vi "Write Subordinate Object Queue.vi"(8 "error in (no error)":errorcluster, 9 "Name":string, 10 "Caller-To-Actor Enqueuer":refnum<class "Message Enqueuer.lvclass">, 11 "Measure Object in":refnum<class "Template Module.lvclass">) -> (0 "error out":errorcluster, 3 "Measure Object out":refnum<class "Template Module.lvclass">)   [LabVIEW 2018, in "Template Module.lvclass"]
uses:
  Template Module.lvclass
  <vilib>/ActorFramework/Message Enqueuer/Message Enqueuer.lvclass
  Template Module.lvclass/Template Module.ctl
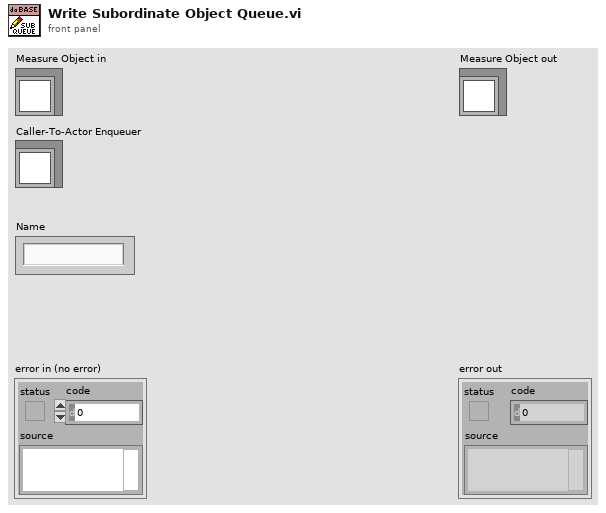
[diagram p1: front panel]
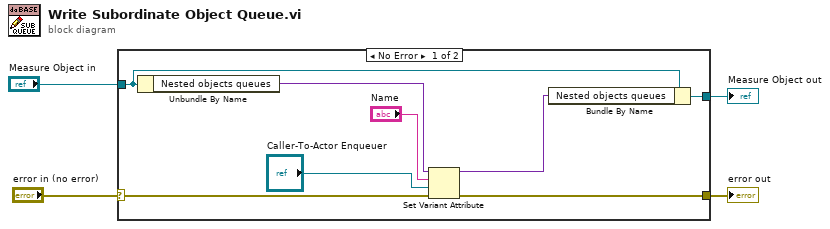
[diagram p0: block diagram]
diagram:
  n1 = case shown="No Error" "error in (no error)" {
    selector: "error in (no error)" -> [w8 w14]
    tunnel: [w5 w14] -> w3
    tunnel: [w7 w13] -> w1
    tunnel: "Measure Object in" -> [w12 w13]
    frame No Error {
      n2 = Unbundle By Name(w12) -> ("Nested objects queues"=w11:variant)
      n3 = Set Variant Attribute(Variant=w11, name="Name", value="Caller-To-Actor Enqueuer", error in=w8) -> (Variant out=w6:variant, error out=w5:errorcluster)  [unwired: 1 out]
      n4 = Bundle By Name(cluster=w12, "Nested objects queues"=w6) -> (w7:refnum<class "Template Module.lvclass">)
    }
    frame Error {
    }
  }
  "error out" <- w3
  "Measure Object out" <- w1
